vi "Outer Product.vi"   [LabVIEW 2020, in "NI_AALBase.lvlib"]
doc: "Computes the outer product of <B>X Vector</B> and <B>Y Vector</B>. The data types you wire to the <B>X Vector</B> and <B>Y Vector</B> inputs determine the polymorphic instance to use."
uses:
  NI_AALBase.lvlib
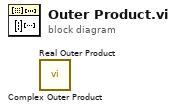
[diagram p0: block diagram]
diagram:
  n1 = call "Complex Outer Product.vi"() -> ()  [unwired: 2 in, 2 out]
  n2 = call "Real Outer Product.vi"() -> ()  [unwired: 2 in, 2 out]
